vi "TcA02-004_AttributesCanBeModifiedFasterThanGOOP1.vi"(1 "Input buffer":T3="1", 3 "Invocation info":T2, 5 "error in (no error)":errorcluster, 6 "Add log to result?":bool) -> (16 "Test Data":T1 {"Numeric Measurement" format="%.2f"}, 19 "error out":errorcluster)   [LabVIEW 2020]
doc: "Test case template."
uses:
  Shared/Support_InputBuffer.ctl
  Shared/Support_InvocationInfo.ctl
  Shared/Support_TestData.ctl
  Shared/Support_ResultType.ctl
  TestClasses/G#BaseClass1_class/G#BaseClass1.lvclass
  <vilib>/addons/_AddQ/G#Object/G#Object.lvclass
panel:
  in  "Test name":string="TcA02-004 Attributes can be modified faster than GOOP1"
  out "Test result":bool
  out "Result":string
  # "Verify that object attributes are modified faster\nthan GOOP1 for an attribute of fixed size."
  # "Sub test case"
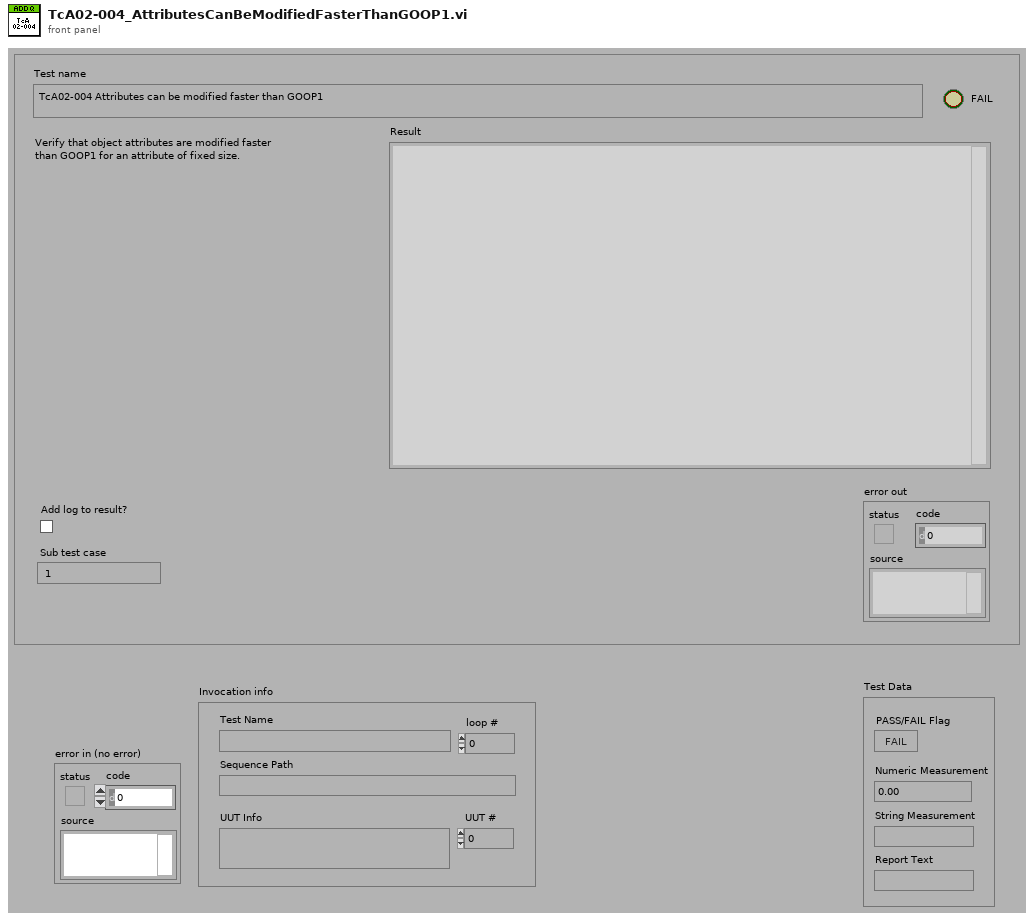
[diagram p1: front panel]
types:
  T1 = typedef "Support_TestData.ctl" = cluster{"PASS/FAIL Flag":bool, "Numeric Measurement":dbl, "String Measurement":string, "Report Text":string}
  T2 = typedef "Support_InvocationInfo.ctl" = cluster{"UUT #":i32, "loop #":i32, "UUT Info":string, "Test Name":string, "Sequence Path":path}
  T3 = typedef "Support_InputBuffer.ctl" = string
  T4 = typedef "Support_ResultType.ctl" = cluster{"Pass":bool, "Comment":string, "MeasurementValue":dbl}
  T5 = typedef "TcOldClass_Object Reference.ctl" = refnum<k1>
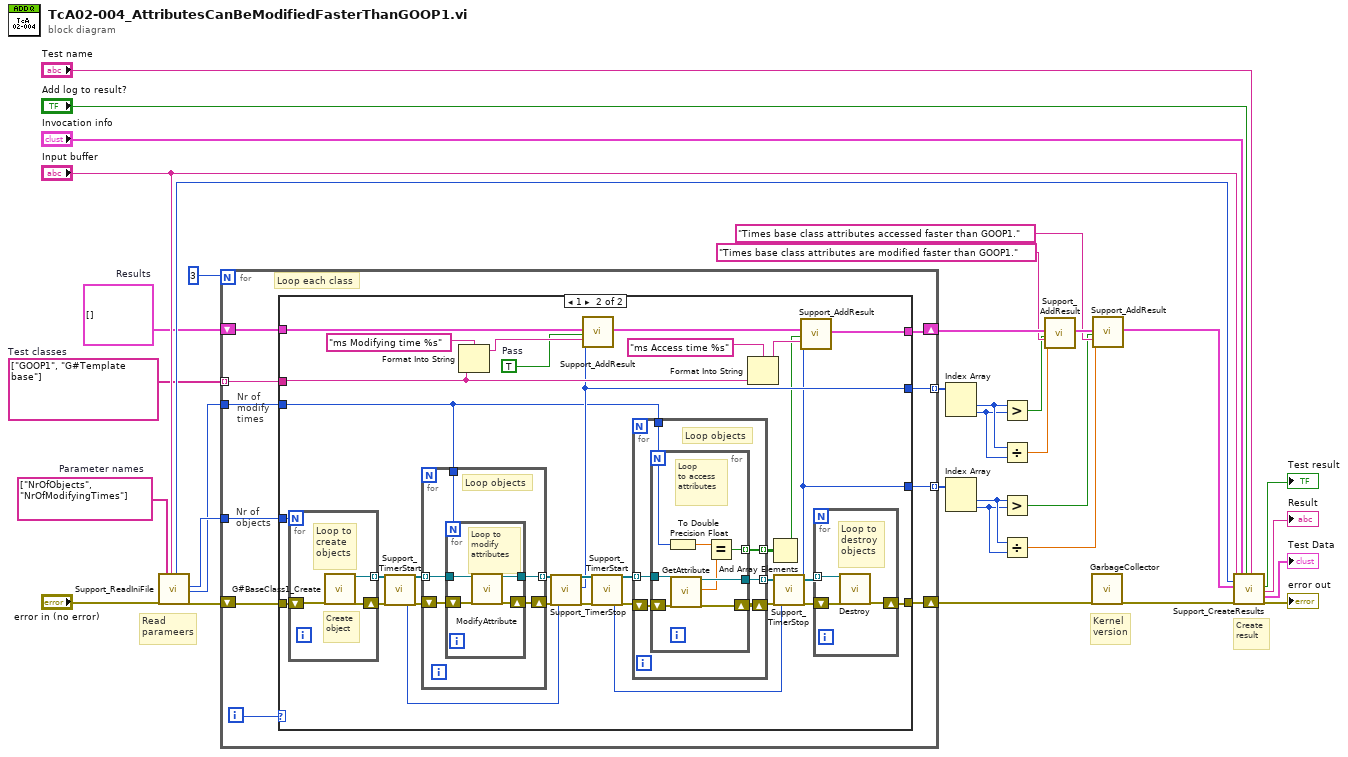
[diagram p0: block diagram]
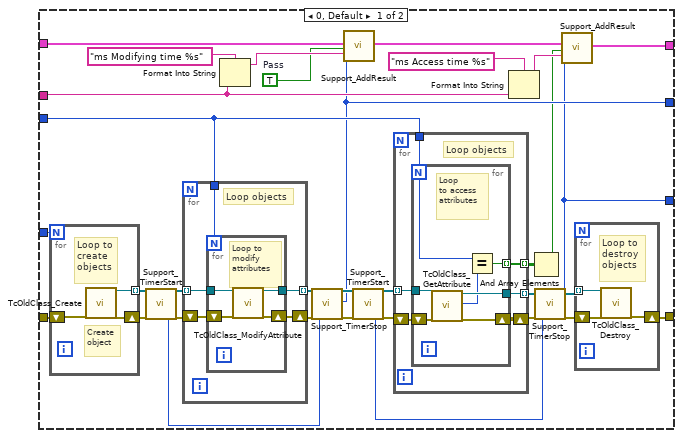
[diagram p2: hidden frame]
diagram:
  w16 = string[] ["GOOP1", "G#Template base"]  # Test classes
  w17 = T4[] []  # Results
  w19 = string[] ["NrOfObjects", "NrOfModifyingTimes"]  # Parameter names
  # "Kernel\nversion"
  # "Read\nparameers"
  # "Create\nresult"
  n1 = call "Support_ReadIniFile.vi"("error in (no error)"="error in (no error)", "Parameter names"=w19, "Sub test case"="Input buffer") -> ("Timer start"=w24:u32, "Parameter1 as I32"=w20:i32, "Parameter2 as I32"=w18:i32, "error out"=w21:errorcluster)  [unwired: 9 in, 4 out]
  n2 = for {
    N: 3 -> [_]
    tunnel: w20 -> [w44]
    shift-right: [w42] -> w22
    shift-left: w21 -> [w41]
    tunnel: w18 -> [w40]
    shift-right: [w37] -> w14
    shift-left: w17 -> [w38]
    tunnel: w16 -> [w39] mode=indexing
    tunnel: [w36] -> w10 mode=indexing
    tunnel: [w35] -> w11 mode=indexing
    i -> [w43]
    # "Nr of\nobjects"
    # "Nr of\nmodify\ntimes"
    # "Loop each class"
    n3 = case shown="1" w43 {
      tunnel: w41 -> [w71 w128]
      tunnel: w44 -> [w73 w130]
      tunnel: [w63 w120] -> w42
      tunnel: w40 -> [w60 w102]
      tunnel: w39 -> [w51 w109]
      tunnel: w38 -> [w57 w115]
      tunnel: [w50 w108] -> w37
      tunnel: [w49 w107] -> w36
      tunnel: [w48 w106] -> w35
      frame 0, Default {
        w46 = TRUE  # Pass
        n4 = for {
          N: w73 -> [_]
          shift-right: [w99] -> w70
          shift-left: w71 -> [w100]
          tunnel: [w101] -> w69 mode=indexing
          # "Create\nobject"
          # "Loop to\ncreate\nobjects"
          n5 = call "TcOldClass_Create.vi"("error in (no error)"=w100) -> ("reference"=w101:T5, "error out"=w99:errorcluster)  [unwired: 17 in]
        }
        n6 = call "Support_TimerStart.vi"("error in (no error)"=w70) -> ("Start time"=w72:u32, "error out"=w68:errorcluster)  [unwired: 17 in]
        n7 = for {
          tunnel: w69 -> [w78] mode=indexing
          tunnel: w60 -> [w77]
          tunnel: [w76] -> w61 mode=indexing
          shift-right: [w74] -> w67
          shift-left: w68 -> [w75]
          # "Loop objects"
          n8 = for {
            N: w77 -> [_]
            shift-right: [w81] -> w74
            shift-left: w75 -> [w82]
            tunnel: w78 -> [w80]
            tunnel: [w79] -> w76
            # "Loop to\nmodify\nattributes"
            n9 = call "TcOldClass_ModifyAttribute.vi"("reference"=w80, "error in (no error)"=w82) -> ("duplicate reference"=w79:T5, "error out"=w81:errorcluster)  [unwired: 15 in, 1 out]
          }
        }
        n10 = Format Into String(format string="ms Modifying time %s", w51) -> (resulting string=w55:string)  [unwired: 2 in, 1 out]
        n11 = call "Support_TimerStop.vi"("error in (no error)"=w67, "Start time"=w72) -> ("Time (ms)"=w49:u32, "error out"=w66:errorcluster)  [unwired: 16 in]
        n12 = call "Support_AddResult.vi"("Results in"=w57, "Pass"=w46, "Comment"=w55, "MeasurementValue"=w49) -> ("Results out"=w54:T4[])  [unwired: 15 in]
        n13 = call "Support_TimerStart.vi"("error in (no error)"=w66) -> ("Start time"=w58:u32, "error out"=w65:errorcluster)  [unwired: 17 in]
        n14 = for {
          shift-right: [w87] -> w64
          shift-left: w65 -> [w88]
          tunnel: w61 -> [w86] mode=indexing
          tunnel: w60 -> [w85]
          tunnel: [w84] -> w59 mode=indexing
          tunnel: [w83] -> w45 mode=indexing
          # "Loop objects"
          n15 = for {
            N: w85 -> [w90]
            shift-right: [w94] -> w87
            shift-left: w88 -> [w95]
            tunnel: w86 -> [w93]
            tunnel: [w92] -> w84
            tunnel: [w89] -> w83 mode=indexing
            # "Loop\nto access\nattributes"
            n16 = call "TcOldClass_GetAttribute.vi"("reference"=w93, "error in (no error)"=w95) -> ("duplicate reference"=w92:T5, "tcRootAttribute"=w91:i32, "error out"=w94:errorcluster)  [unwired: 13 in, 2 out]
            n17 = Equal?(x=w90, y=w91) -> (x = y?=w89:bool)
          }
        }
        n18 = Format Into String(format string="ms Access time %s", w51) -> (resulting string=w53:string)  [unwired: 2 in, 1 out]
        n19 = And Array Elements(Boolean array=w45) -> (logical AND=w47:bool)
        n20 = call "Support_TimerStop.vi"("error in (no error)"=w64, "Start time"=w58) -> ("Time (ms)"=w48:u32, "error out"=w62:errorcluster)  [unwired: 16 in]
        n21 = call "Support_AddResult.vi"("Results in"=w54, "Pass"=w47, "Comment"=w53, "MeasurementValue"=w48) -> ("Results out"=w50:T4[])  [unwired: 15 in]
        n22 = for {
          tunnel: w59 -> [w98] mode=indexing
          shift-right: [w96] -> w63
          shift-left: w62 -> [w97]
          # "Loop to \ndestroy\nobjects"
          n23 = call "TcOldClass_Destroy.vi"("reference"=w98, "error in (no error)"=w97) -> ("error out"=w96:errorcluster)  [unwired: 17 in]
        }
      }
      frame 1 {
        w104 = TRUE  # Pass
        n24 = for {
          N: w130 -> [_]
          shift-right: [w158] -> w127
          shift-left: w128 -> [w159]
          tunnel: [w157] -> w126 mode=indexing
          # "Create\nobject"
          # "Loop to\ncreate\nobjects"
          n25 = call "G#BaseClass1_Create.vi"("error in (no error)"=w159) -> ("reference out"=w157:refnum<class "G#BaseClass1.lvclass">, "error out"=w158:errorcluster)  [unwired: 16 in, 1 out]
        }
        n26 = call "Support_TimerStart.vi"("error in (no error)"=w127) -> ("Start time"=w129:u32, "error out"=w125:errorcluster)  [unwired: 17 in]
        n27 = for {
          tunnel: w126 -> [w135] mode=indexing
          tunnel: w102 -> [w134]
          tunnel: [w133] -> w118 mode=indexing
          shift-right: [w131] -> w124
          shift-left: w125 -> [w132]
          # "Loop objects"
          n28 = for {
            N: w134 -> [_]
            shift-right: [w138] -> w131
            shift-left: w132 -> [w139]
            tunnel: w135 -> [w137]
            tunnel: [w136] -> w133
            # "Loop to\nmodify\nattributes"
            n29 = call-dynamic "ModifyAttribute.vi"("reference in"=w137, "error in (no error)"=w139) -> ("reference out"=w136:refnum<class "G#BaseClass1.lvclass">, "error out"=w138:errorcluster)  [unwired: 16 in]
          }
        }
        n30 = Format Into String(format string="ms Modifying time %s", w109) -> (resulting string=w113:string)  [unwired: 2 in, 1 out]
        n31 = call "Support_TimerStop.vi"("error in (no error)"=w124, "Start time"=w129) -> ("Time (ms)"=w107:u32, "error out"=w123:errorcluster)  [unwired: 16 in]
        n32 = call "Support_AddResult.vi"("Results in"=w115, "Pass"=w104, "Comment"=w113, "MeasurementValue"=w107) -> ("Results out"=w112:T4[])  [unwired: 15 in]
        n33 = call "Support_TimerStart.vi"("error in (no error)"=w123) -> ("Start time"=w116:u32, "error out"=w122:errorcluster)  [unwired: 17 in]
        n34 = for {
          shift-right: [w144] -> w121
          shift-left: w122 -> [w145]
          tunnel: w118 -> [w143] mode=indexing
          tunnel: w102 -> [w142]
          tunnel: [w141] -> w117 mode=indexing
          tunnel: [w140] -> w103 mode=indexing
          # "Loop objects"
          n35 = for {
            N: w142 -> [w148]
            shift-right: [w152] -> w144
            shift-left: w145 -> [w153]
            tunnel: w143 -> [w151]
            tunnel: [w150] -> w141
            tunnel: [w147] -> w140 mode=indexing
            # "Loop\nto access\nattributes"
            n36 = To Double Precision Float(number=w148) -> (double precision float=w146:dbl)
            n37 = call-dynamic "GetAttribute.vi"("reference in"=w151, "error in (no error)"=w153) -> ("reference out"=w150:refnum<class "G#BaseClass1.lvclass">, "Numeric"=w149:dbl, "error out"=w152:errorcluster)  [unwired: 14 in, 1 out]
            n38 = Equal?(x=w146, y=w149) -> (x = y?=w147:bool)
          }
        }
        n39 = Format Into String(format string="ms Access time %s", w109) -> (resulting string=w111:string)  [unwired: 2 in, 1 out]
        n40 = And Array Elements(Boolean array=w103) -> (logical AND=w105:bool)
        n41 = call "Support_TimerStop.vi"("error in (no error)"=w121, "Start time"=w116) -> ("Time (ms)"=w106:u32, "error out"=w119:errorcluster)  [unwired: 16 in]
        n42 = call "Support_AddResult.vi"("Results in"=w112, "Pass"=w105, "Comment"=w111, "MeasurementValue"=w106) -> ("Results out"=w108:T4[])  [unwired: 15 in]
        n43 = for {
          tunnel: w117 -> [w156] mode=indexing
          shift-right: [w154] -> w120
          shift-left: w119 -> [w155]
          # "Loop to \ndestroy\nobjects"
          n44 = call-dynamic "Destroy.vi"("reference in"=w156, "error in (no error)"=w155) -> ("error out"=w154:errorcluster)  [unwired: 16 in, 1 out]
        }
      }
    }
  }
  n45 = Index Array(array=w10) -> (element #1=w9:u32, element #2=w7:u32)  [unwired: 2 in]
  n46 = Index Array(array=w11) -> (element #1=w8:u32, element #2=w6:u32)  [unwired: 2 in]
  n47 = Greater?(x=w9, y=w7) -> (0:w5:bool)
  n48 = Divide(x=w9, y=w7) -> (x/y=w4:dbl)
  n49 = Greater?(x=w8, y=w6) -> (0:w3:bool)
  n50 = Divide(x=w8, y=w6) -> (x/y=w2:dbl)
  n51 = call "Support_AddResult.vi"("Results in"=w14, "Pass"=w5, "Comment"="Times base class attributes are modified faster than GOOP1.", "MeasurementValue"=w4) -> ("Results out"=w15:T4[])  [unwired: 15 in]
  n52 = call <vilib>:"GarbageCollector.vi"("error in (no error)"=w22) -> ("error out"=w26:errorcluster)  [unwired: 16 in, 2 out]
  n53 = call "Support_AddResult.vi"("Results in"=w15, "Pass"=w3, "Comment"="Times base class attributes accessed faster than GOOP1.", "MeasurementValue"=w2) -> ("Results out"=w1:T4[])  [unwired: 15 in]
  n54 = call "Support_CreateResults.vi"("Sub test case"="Input buffer", "Timer start"=w24, "Results"=w1, "error in (no error)"=w26, "Invocation info"="Invocation info", "Add log to result?"="Add log to result?", "Test name"="Test name") -> ("Pass/fail flag"=→"Test result":bool, "Result"=→"Result":string, "Test Data"=→"Test Data":T1, "error out"=→"error out":errorcluster)  [unwired: 9 in]
